vi "Untitled 3 (SubVI).vi"(10 "Numeric 3":i32, 11 "Array":dbl[](array[numeric])) -> (1 "Boolean":bool, 2 "Numeric":dbl, 3 "element":dbl, 4 "Corrente":dbl, 5 "Field":dbl, 6 "todo":dbl[](array[numeric]), 7 "RELE":bool)   [LabVIEW 2015]
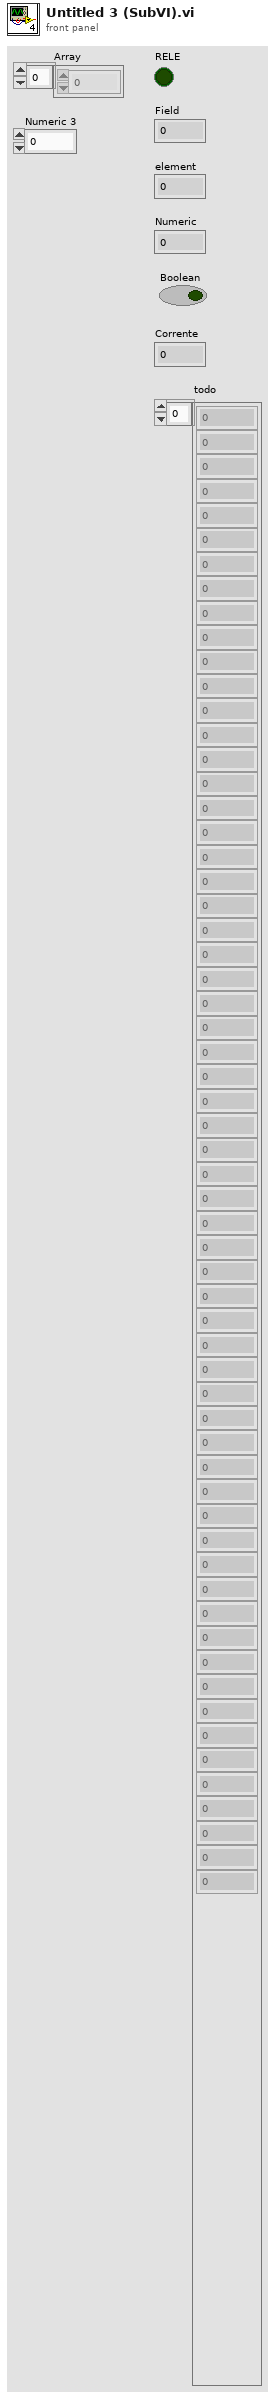
[diagram p1: front panel]
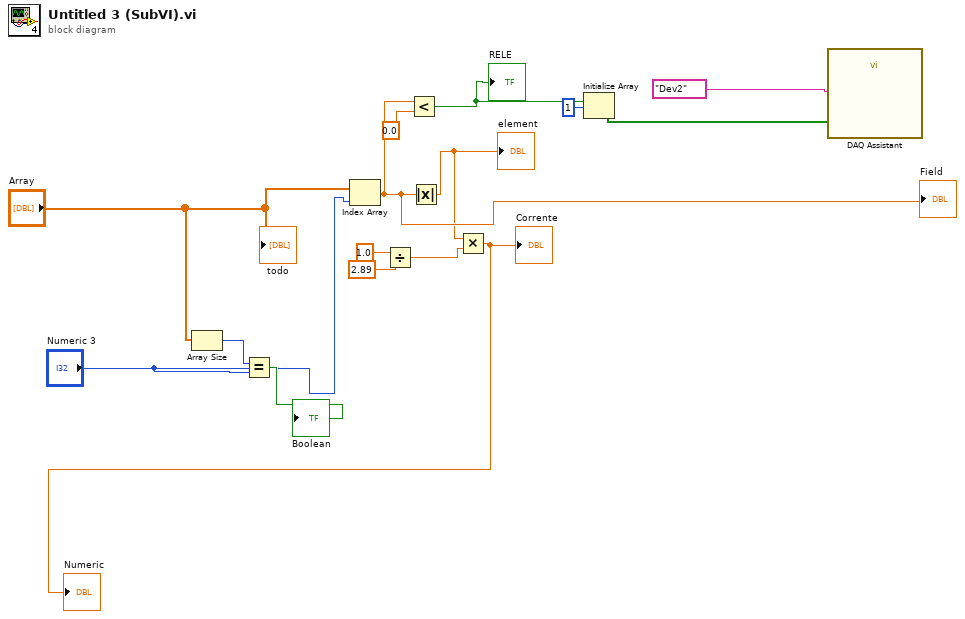
[diagram p0: block diagram]
diagram:
  n1 = Array Size(array="Array") -> (size(s)=w13:i32)
  n2 = Equal?(x=w13, y="Numeric 3") -> (x = y?=→"Boolean":bool)
  n3 = Index Array(array="Array", index="Numeric 3") -> (element=w12:dbl)
  "Field" <- w12
  n4 = Divide(x=1.0, y=2.89) -> (x/y=w4:dbl)
  n5 = Less?(x=w12, y=0.0) -> (x < y?=w7:bool)
  "RELE" <- w7
  n6 = Absolute Value(x=w12) -> (abs(x)=w11:dbl)
  "element" <- w11
  n7 = Multiply(x=w11, y=w4) -> (x*y=→"Corrente" →"Numeric":dbl)
  n8 = Initialize Array(w7, 1 ("dimension size")) -> (w9:bool[])
  n9 = call "DAQ Assistant"("data"=w9, "device name"=tag "Dev2") -> ()  [unwired: 16 in, 2 out]
  "todo" <- "Array"
